vi "Fail.vi"(7 "Description":string, 8 "error in (no error)":errorcluster, 9 "Message":string, 11 "LUnit Test Case In":refnum<class "LUnit Inheriting Test Case.lvclass">) -> (0 "error out":errorcluster, 3 "LUnit Test Case Out":refnum<class "LUnit Inheriting Test Case.lvclass">)   [LabVIEW 2020]
doc: "Generates a fail result for the calling test method. A description and message may be provided."
uses:
  LUnit Inheriting Test Case.lvclass/LUnit Inheriting Test Case.ctl
  Core/Result/Type.ctl
  Core/Result/Result.lvlib
  LUnit Inheriting Test Case.lvclass
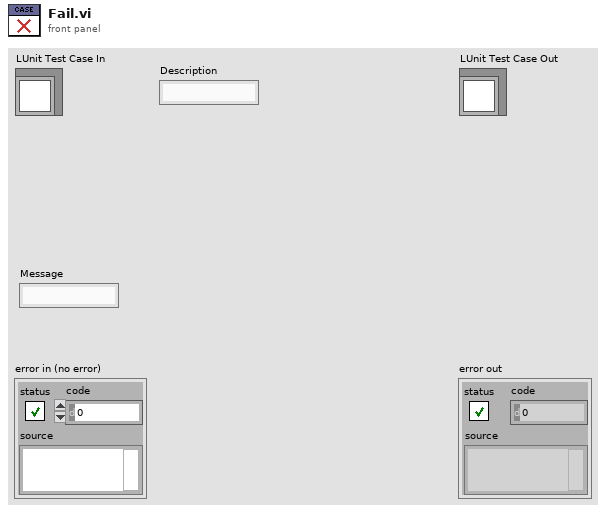
[diagram p1: front panel]
types:
  T1 = typedef "Result.lvlib/Type.ctl" = enum16{"Test Case", "Test Suite", "Test Run", "Pass", "Fail", "Skip", "Pass if", "Fail if", "Pass if Error", "Fail if Error", "Pass if Equal", "Fail if Equal"}
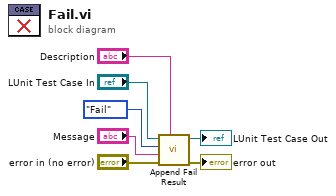
[diagram p0: block diagram]
diagram:
  n1 = call "Append Fail Result.vi"("Description"="Description", "error in (no error)"="error in (no error)", "Message"="Message", "Result Type"=Type."Fail", "LUnit Test Case In"="LUnit Test Case In") -> ("error out"=→"error out":errorcluster, "LUnit Test Case Out"=→"LUnit Test Case Out":refnum<class "LUnit Inheriting Test Case.lvclass">)  [unwired: 5 in]
